vi "refMgr_Example5.vi"() -> ()   [LabVIEW 2017]
uses:
  9c7bb58b-32f4-4c77-afc8-e3433cf93365.vi
  9c7bb58b-32f4-4c77-afc8-e3433cf93365.vi/1b47866c-8e2d-43a7-815f-8cf18635e5a1.vi
  <userlib>/_NEVSTOP/TagDB/_Support/Change Detector/TagDB dbChanged.vi
  <userlib>/_NEVSTOP/TagDB/_Support/Error/_Clear Errors.vi
  9c7bb58b-32f4-4c77-afc8-e3433cf93365.vi/1b47866c-8e2d-43a7-815f-8cf18635e5a1.vi/29b2ea6d-6d7f-4e4a-ad31-a5cb760462c7.vi
  <userlib>/_NEVSTOP/TagDB/API/TagDB-Status.vi
  <userlib>/_NEVSTOP/TagDB/_Support/Change Detector/TagDB ChangeFlag.vi
  <userlib>/_NEVSTOP/TagDB/_Support/DataAccess/_NameCacher.vi
  <userlib>/_NEVSTOP/TagDB/_Support/Error/_[error50002]Invalid DataType.vi
  <userlib>/_NEVSTOP/TagDB/_Support/Error/_[error50000]Invalid DB REF.vi
  <userlib>/_NEVSTOP/TagDB/_Support/DataAccess/TagDB Ref to DVR.vi
  <userlib>/_NEVSTOP/TagDB/_Support/URL/TRIM-BOTH-SPACE.vi
  <userlib>/_NEVSTOP/TagDB/_Support/Error/_Build Error Cluster.vi
  RefManager/TagDB RefManager.lvlib
  <userlib>/_NEVSTOP/TagDB/TagDB.lvlib
panel:
  out "names":string[](array[string])
  in  "Color Box":u32(colorbox)
  # "asdfasdf"
  # "asdfqwefvcq"
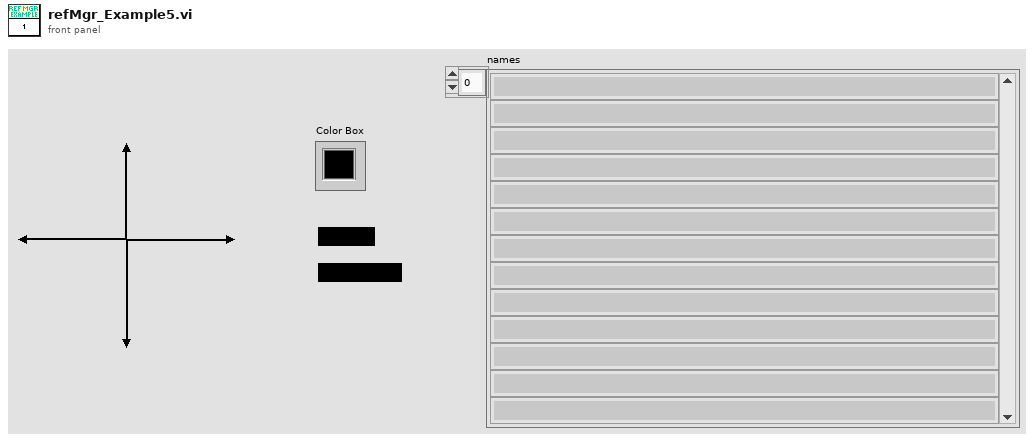
[diagram p1: front panel]
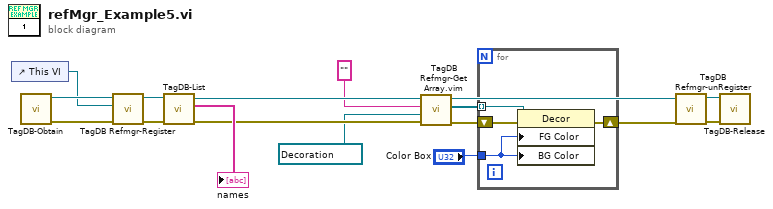
[diagram p0: block diagram]
diagram:
  n1 = control-ref of="This VI"() -> (w11:refnum<vi>)
  n2 = call <userlib>:"TagDB-Obtain.vi"() -> ("error out"=w15:errorcluster, "TagDB"=w17:refnum<k1>)  [unwired: 5 in, 1 out]
  n3 = call "TagDB Refmgr-Register.vi"("error in (no error)"=w15, "VI Refnum"=w11, "TagDB in"=w17) -> ("error out"=w14:errorcluster, "TagDB out"=w16:refnum<k1>)  [unwired: 6 in, 1 out]
  n4 = call <userlib>:"TagDB-List.vi"("error in (no error)"=w14, "TagDB"=w16) -> ("error out"=w8:errorcluster, "names"=→"names":string[], "TagDB(dup)"=w9:refnum<k1>)  [unwired: 6 in, 1 out]
  n5 = call "TagDB Refmgr-Get Array.vim"("error in (no error)"=w8, "Type"=refnum<vi> refnum, "RegExp"="", "DB Ref"=w9) -> ("error out"=w7:errorcluster, "References"=w2:refnum<vi>[], "DB Ref(dup)"=w6:refnum<k1>)  [unwired: 4 in, 1 out]
  n6 = for {
    tunnel: w2 -> [w19] mode=indexing
    shift-right: [w20] -> w3
    shift-left: w7 -> [w21]
    tunnel: "Color Box" -> [w18]
    n7 = property class="Decor"(reference=w19, error in=w21, "FG Color"=w18, "BG Color"=w18) -> (error out=w20:errorcluster)  [unwired: 1 out]
  }
  n8 = call "TagDB Refmgr-unRegister.vi"("error in (no error)"=w3, "TagDB in"=w6) -> ("error out"=w12:errorcluster, "TagDB out"=w13:refnum<k1>)  [unwired: 8 in]
  n9 = call <userlib>:"TagDB-Release.vi"("error in (no error)"=w12, "TagDB"=w13) -> ()  [unwired: 9 in, 1 out]
